vi "Read Humidity and Temperature.vi"(8 "error in (no error)":errorcluster) -> (0 "error out":errorcluster, 1 "temperature (°C)":u8, 2 "humidity (%)":u8, 3 "refnum out":refnum<k20>)   [LabVIEW 2015]
uses:
  <vilib>/rvi/interface/nirviReadWriteControl/nirviReadWriteControl.xnode
  NiFpgaLv.dll
  <vilib>/Utility/error.llb/Error Cluster From Error Code.vi
  <vilib>/rvi/interface/Simulation/niFpgaSimulationCallBeginRW.vi
  <vilib>/rvi/errors/niLvFpgaAdjustHostInterfaceError.vi
  <vilib>/rvi/interface/nirviOpenFPGA/nirviOpenFPGA.xnode
  <vilib>/userdefined/High Color/nirio_resource_hc.ctl
  <vilib>/myRIO/Instrument Drivers/Onboard IO/DIO/DIO.lvlib
  <vilib>/FPGAPlugInAG/myRIO-1900/niLvFpga_Open_myRIO-1900.vi
  <vilib>/rvi/interface/common/dynamic/niFpgaDynamicAddResources.vi
  <vilib>/myRIO/Common/Instrument Driver Framework/Utilities/typedefs/FPGA Ref Manager Action Enum.ctl
  FPGA Bitfiles/IoTFoundationDEM_FPGATarget_DHT11(FPGA)_nBL-L-qrK6U.lvbitx
  Sensor2.ctl
  <vilib>/myRIO/Instrument Drivers/Onboard Devices/Accelerometer/Accelerometer.lvlib
  <vilib>/myRIO/Common/Instrument Driver Framework/myRIO v1.0/Accelerometer/typedefs/Accelerometer FPGA Reference.ctl
  <vilib>/myRIO/Common/Instrument Driver Framework/myRIO v1.0/Accelerometer/typedefs/Accelerometer Channels Enum.ctl
  <vilib>/myRIO/Common/Instrument Driver Framework/myRIO v1.0/Accelerometer/typedefs/Accelerometer Channels List.ctl
  <vilib>/myRIO/Common/Instrument Driver Framework/Utilities/typedefs/Generic FPGA Reference.ctl
  <vilib>/myRIO/Common/Instrument Driver Framework/Utilities/typedefs/myRIO v1.0 Reference.ctl
  <vilib>/myRIO/Common/Instrument Driver Framework/Utilities/typedefs/Hardware Version Enum.ctl
  <vilib>/myRIO/Common/Instrument Driver Framework/Utilities/typedefs/myRIO Generic Hardware Reference.ctl
  <vilib>/myRIO/Instrument Drivers/Onboard Devices/Accelerometer/typedefs/Accelerometer Reference.ctl
  <vilib>/myRIO/Instrument Drivers/Onboard Devices/Accelerometer/vis/myRIO Accelerometer Open.xnode
  <vilib>/myRIO/Common/Instrument Driver Framework/myRIO v1.0/Accelerometer/vis/myRIO v1.1 Open Accelerometer.vi
  <vilib>/myRIO/Common/Instrument Driver Framework/myRIO v1.0/DIO/typedefs/DIO Channels Enum.ctl
  <vilib>/myRIO/Common/Instrument Driver Framework/myRIO v1.0/DIO/typedefs/DIO Channels List.ctl
  <vilib>/myRIO/Instrument Drivers/Onboard IO/DIO/typedefs/DIO Reference.ctl
panel:
  in  "DIO Ref In":T1
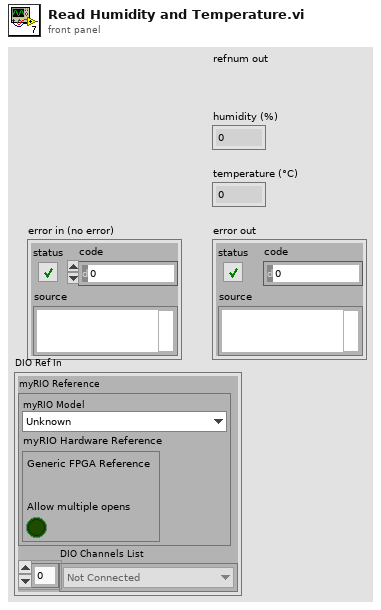
[diagram p1: front panel]
types:
  T1 = typedef "DIO.lvlib/DIO Reference.ctl" = cluster{"myRIO Reference":T2, "DIO Channels List":T6}
  T2 = typedef "myRIO Generic Hardware Reference.ctl" = cluster{"myRIO Model":T3, "myRIO Hardware Reference":T4}
  T3 = typedef "Hardware Version Enum.ctl" = enum16{"Unknown", "myRIO-1900", "myRIO-1950", "roboRIO"}
  T4 = typedef "myRIO v1.0 Reference.ctl" = cluster{"Generic FPGA Reference":T5, "Allow multiple opens":bool}
  T5 = typedef "Generic FPGA Reference.ctl" = refnum<k20>
  T6 = typedef "DIO Channels List.ctl" = T7[]
  T7 = typedef "DIO Channels Enum.ctl" = enum16{"Not Connected", "C/DIO0", "C/DIO1", "C/DIO2", "C/DIO3", "C/DIO4", "C/DIO5", "C/DIO6", "C/DIO7", "A/DIO0", "A/DIO1", "A/DIO2", "A/DIO3", "A/DIO4", "A/DIO5", "A/DIO6", "A/DIO7", "A/DIO8", "A/DIO9", "A/DIO10", "A/DIO11", "A/DIO12", "A/DIO13", "A/DIO14", "A/DIO15", "B/DIO0", "B/DIO1", "B/DIO2", "B/DIO3", "B/DIO4", "B/DIO5", "B/DIO6", "B/DIO7", "B/DIO8", "B/DIO9", "B/DIO10", "B/DIO11", "B/DIO12", "B/DIO13", "B/DIO14", "B/DIO15", "LED0", "LED1", "LED2", "LED3", "Button0", "DIO/DIO0", "DIO/DIO1", "DIO/DIO2", "DIO/DIO3", "DIO/DIO4", "DIO/DIO5", "DIO/DIO6", "DIO/DIO7", "DIO/DIO8", "DIO/DIO9", "SPI/CS0", "SPI/CS1", "SPI/CS2", "SPI/CS3", "LED RADIO (Green)", "LED RADIO (Red)", "LED COMM (Green)", "LED COMM (Red)", "LED MODE (Green)", "LED MODE (Red)"}
  T8 = typedef "Accelerometer FPGA Reference.ctl" = refnum<k20>
  T9 = typedef "nirio_resource_hc.ctl" = tag
  T10 = typedef "Sensor2.ctl" = refnum<k20>
  T11 = typedef "FPGA Ref Manager Action Enum.ctl" = enum16{"Get", "Set", "Reset"}
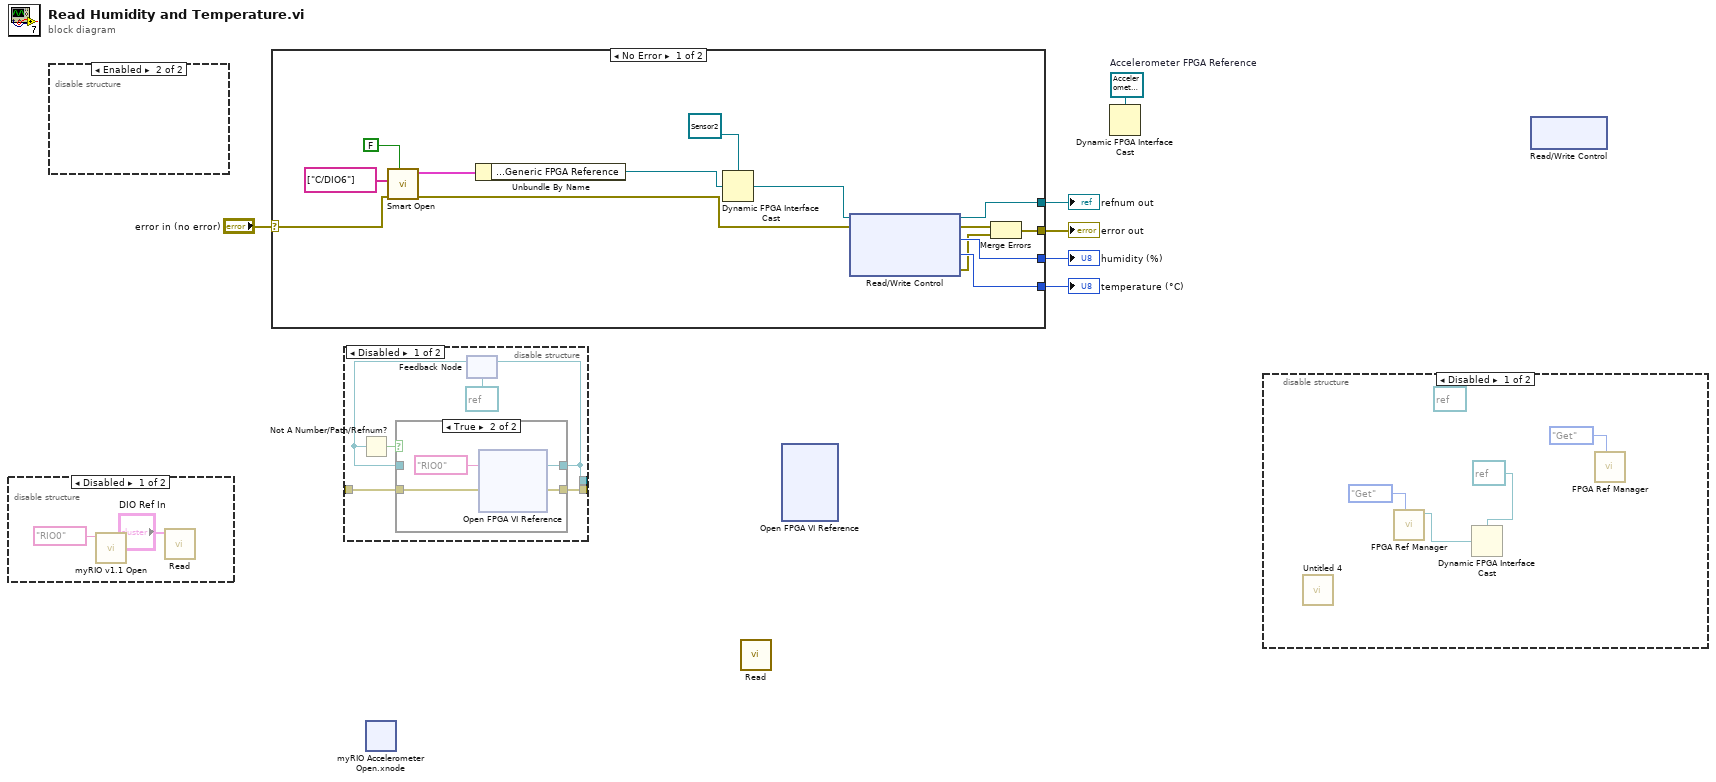
[diagram p0: block diagram]
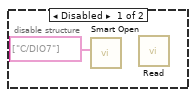
[diagram p4: hidden frame]
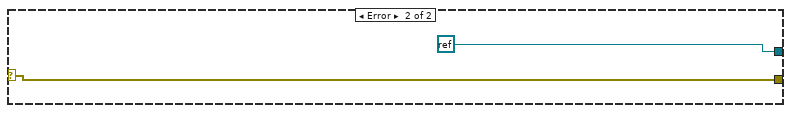
[diagram p7: hidden frame]
diagram:
  w1 = T8 refnum  # Accelerometer FPGA Reference
  n1 = disable-structure shown="Disabled" {
    frame Disabled {
      n2 = call <vilib>:"myRIO v1.1 Open.vi"("Resource name"=T9 "RIO0") -> ()  [unwired: 9 in, 2 out]
      n3 = call <vilib>:"Read.vi"("DIO Ref In"="DIO Ref In") -> ()  [unwired: 8 in, 3 out]
    }
    frame Enabled {
    }
  }
  n4 = disable-structure shown="Enabled" {
    frame Disabled {
      n5 = call <vilib>:"Smart Open.vi"("Channel Names"=tag[] ["C/DIO7"]) -> ()  [unwired: 9 in, 2 out]
      n6 = call <vilib>:"Read.vi"() -> ()  [unwired: 9 in, 3 out]
    }
    frame Enabled {
    }
  }
  n7 = case shown="No Error" "error in (no error)" {
    selector: "error in (no error)" -> [w12 w25]
    tunnel: [w23 _] -> w6
    tunnel: [w22 _] -> w5
    tunnel: [w21 refnum<k0> refnum] -> w4
    tunnel: [w20 w25] -> w3
    frame No Error {
      n8 = call <vilib>:"Smart Open.vi"("Allow multiple opens?"=FALSE, "error in (no error)"=w12, "Channel Names"=tag[] ["C/DIO6"]) -> ("error out"=w13:errorcluster, "DIO Ref Out"=w17:T1)  [unwired: 7 in]
      n9 = Unbundle By Name(w17) -> ("myRIO Reference.myRIO Hardware Reference.Generic FPGA Reference"=w15:T5)
      n10 = Dynamic FPGA Interface Cast(Session In=T10 refnum ("FPGA VI Reference Out"), Type=w15) -> (Session Out=w14:T10)
      n11 = xnode "Read/Write Control"("FPGA VI Reference In"=w14, "error in"=w13) -> ("FPGA VI Reference Out"=w21:T10, "error out"=w18:errorcluster, "Humidity (%)"=w22:u8, "Temperature (°C)"=w23:u8, "error out"=w19:errorcluster)
      n12 = Merge Errors(w18, w19) -> (w20:errorcluster)
    }
    frame Error {
    }
  }
  "temperature (°C)" <- w6
  "humidity (%)" <- w5
  "refnum out" <- w4
  "error out" <- w3
  n13 = disable-structure shown="Disabled" {
    disable-tunnel: [w28 _] -> _
    disable-tunnel: [w27 _] -> _
    disable-tunnel: _ -> [w26 _]
    frame Disabled {
      n14 = feedback #1(refnum<k20> refnum ("FPGA VI Reference Out")) -> (w30:refnum<k20>)
      n15 = Not A Number/Path/Refnum?(number/path/refnum=w30) -> (NaN/Path/Refnum?=w29:bool)
      n16 = case shown="True" w29 {
        tunnel: [w33 w36] -> w28
        tunnel: [w32 w35] -> w27
        tunnel: w26 -> [w32 w34]
        tunnel: w30 -> [w33 _]
        frame False {
        }
        frame True {
          n17 = xnode "Open FPGA VI Reference"("error in"=w34, "resource name"=tag "RIO0") -> ("FPGA VI Reference Out"=w36:refnum<k20>, "error out"=w35:errorcluster)
        }
      }
      n18 = feedback-in #1(w28) -> ()
    }
    frame Enabled {
    }
  }
  n19 = xnode "myRIO Accelerometer Open.xnode"() -> ()  [unwired: 3 in, 2 out]
  n20 = call <vilib>:"Read.vi"() -> ()  [unwired: 9 in, 3 out]
  n21 = xnode "Open FPGA VI Reference"() -> ()  [unwired: 2 in, 2 out]
  n22 = Dynamic FPGA Interface Cast(Session In=w1) -> ()  [unwired: 1 in, 1 out]
  n23 = disable-structure shown="Disabled" {
    frame Disabled {
      w45 = refnum<k20> refnum ("FPGA VI Reference Out")
      n24 = call "Untitled 4.vi"() -> ()  [unwired: 10 in, 2 out]
      n25 = call <vilib>:"FPGA Ref Manager.vi"("Action"=FPGA_Ref_Manager_Action_Enum."Get") -> ("error out"=w43:errorcluster, "Generic FPGA Reference out"=w41:T5, "error in (no error)"=w44:errorcluster)  [unwired: 7 in]
      n26 = Dynamic FPGA Interface Cast(Session In=refnum<k20> refnum ("FPGA VI Reference Out"), Type=w41) -> (Session Out=w42:refnum<k20>)
      n27 = call <vilib>:"FPGA Ref Manager.vi"("Action"=FPGA_Ref_Manager_Action_Enum."Get") -> ()  [unwired: 8 in, 2 out]
    }
    frame Enabled {
    }
  }
  n28 = xnode "Read/Write Control"() -> ()  [unwired: 2 in, 3 out]
